vi "TimeUiTest.vi"() -> ()   [LabVIEW 2018, in "Ui.lvlib"]
uses:
  Ui.lvlib
  Time/Loop.xctl
  Frequency.xctl
panel:
  out "Frequency":i64(xcontrol)
  out "Time (ms)":i64
  out "Loop":T1(xcontrol)
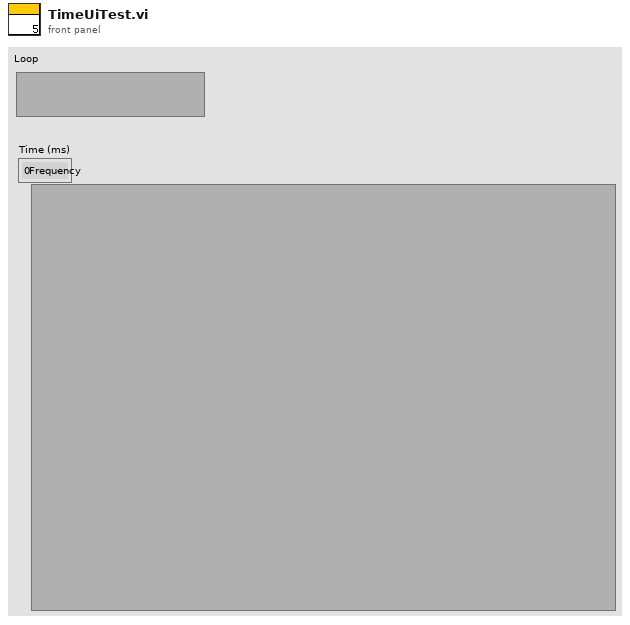
[diagram p1: front panel]
types:
  T1 = cluster{"Cycle":i32, "Status":bool, "Late":bool, "Error":bool, "Time":dbl}
  T2 = cluster{"Stop":bool, "Start":bool, "Time (ms)":i64}
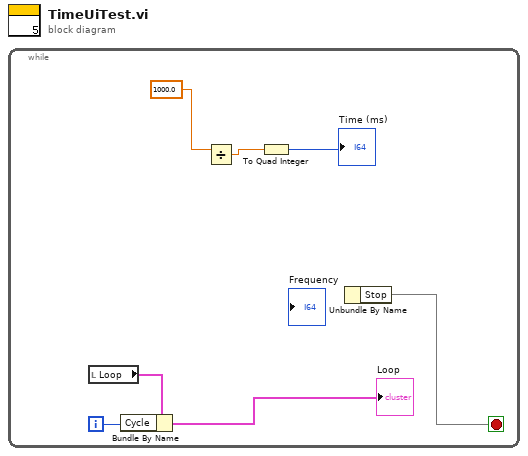
[diagram p0: block diagram]
diagram:
  n1 = while {
    i -> [w8]
    stop <- w6 stop-if-true
    n2 = local read "Loop"() -> (w9:T1)
    n3 = Bundle By Name(cluster=w9, "Cycle"=w8) -> (→"Loop":T1)
    n4 = Divide(x=1000.0) -> (y=w4:dbl, x/y=w2:dbl)
    n5 = To Quad Integer(1:w2) -> (0:→"Time (ms)":i64)
    n6 = Unbundle By Name() -> (w5:T2, "Stop"=w6)
  }
